vi "support.read__multiline_string.vi"(8 "error in (no error)":errorcluster, 11 "table_names":string) -> (0 "error out":errorcluster, 3 "lines":string[](array[string]))   [LabVIEW 2020, in "toml_edit.lvlib"]
uses:
  toml_edit.lvlib
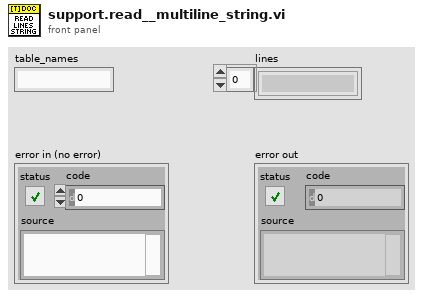
[diagram p1: front panel]
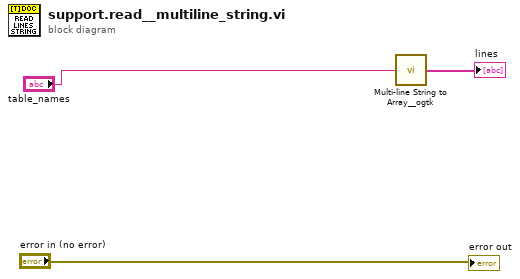
[diagram p0: block diagram]
diagram:
  n1 = call <userlib>:"Multi-line String to Array__ogtk.vi"("string"="table_names") -> ("lines"=→"lines":string[])
  "error out" <- "error in (no error)"
